vi "Init Transport.vi"() -> (3 "Event Transport out":refnum<class "Event Transport.lvclass">)   [LabVIEW 2020, in "jettl.lvlib" / "Event Transport.lvlib" / "Event Transport.lvclass"]
uses:
  Event Transport.lvclass
  Event Transport.lvclass/Event Transport.ctl
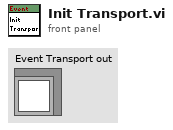
[diagram p1: front panel]
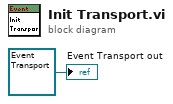
[diagram p0: block diagram]
diagram:
  "Event Transport out" <- refnum<class "Event Transport.lvclass"> refnum ("Event Transport out")
